vi "RunEntuse.vi"() -> ()   [LabVIEW 2012]
uses:
  <vilib>/addons/database/Connection.llb/DB Tools Open Connec (Path).vi
  <vilib>/addons/database/Connection.llb/Conn Execute.vi
  <vilib>/addons/database/Recordset.llb/Rec Fetch Recordset Data (R).vi
  <vilib>/addons/database/Recordset.llb/Rec Destroy - Connection.vi
  <vilib>/addons/database/Recordset.llb/Rec Fetch Integer Data (R).vi
  <vilib>/addons/database/_DB Variant To Data/Database Variant To Data.xnode
  <vilib>/addons/database/NI_Database_API.lvlib
panel:
  out "data 3":string
  out "data 2":string
  out "x > y?":bool
  out "concatenated string":string
  out "data":string
  out "error out":errorcluster
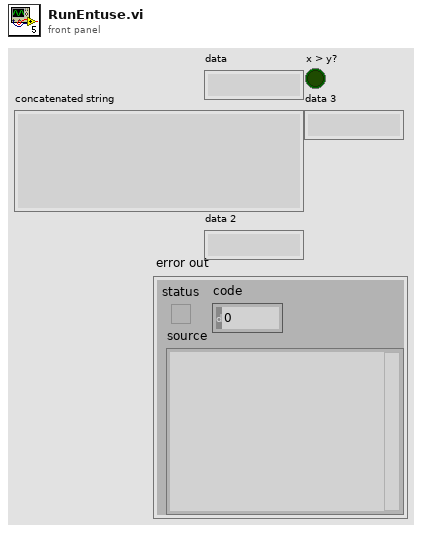
[diagram p1: front panel]
types:
  T1 = typedef "NI_Database_API.lvlib/Conn ObjectReference.ctl" = refnum<k1>
  T2 = typedef "NI_Database_API.lvlib/Rec ObjectReference.ctl" = refnum<k1>
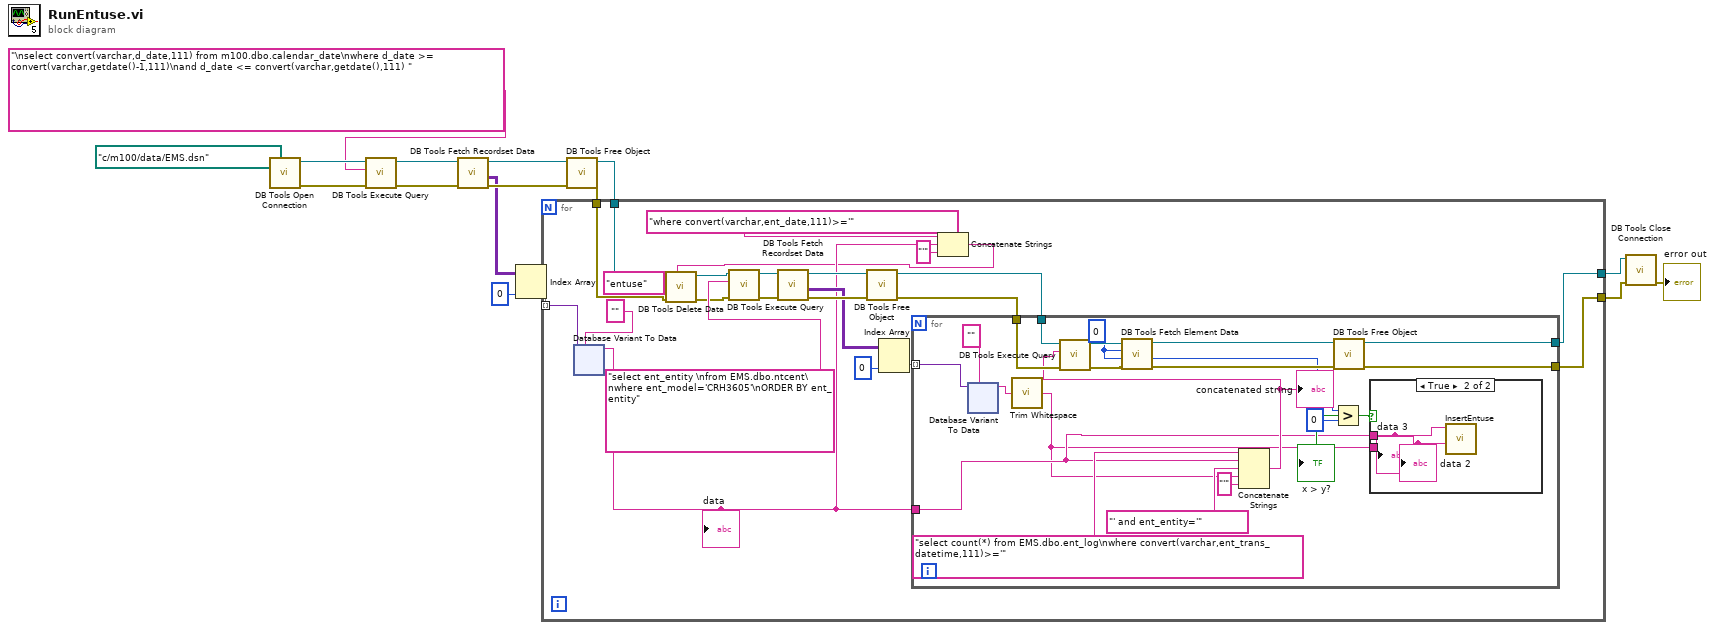
[diagram p0: block diagram]
diagram:
  n1 = call-poly <vilib>:"DB Tools Open Connection.vi"("connection information"=path "c:/m100/data/EMS.dsn") -> ("error out"=w12:errorcluster, "connection reference"=w15:T1)  [unwired: 7 in]
  n2 = call-poly <vilib>:"DB Tools Execute Query.vi"("error in (no error)"=w12, "SQL query"="\nselect convert(varchar,d_date,111) from m100.dbo.calendar_date\nwhere d_date >= convert(varchar,getdate()-1,111)\nand d_date <= convert(varchar,getdate(),111) " ("string"), "connection reference"=w15) -> ("error out"=w11:errorcluster, "recordset reference"=w14:T2)  [unwired: 5 in]
  n3 = call-poly <vilib>:"DB Tools Fetch Recordset Data.vi"("error in (no error)"=w11, "recordset reference"=w14) -> ("error out"=w10:errorcluster, "recordset data"=w7:variant[][], "recordset reference out"=w13:T2)  [unwired: 3 in]
  n4 = Index Array(array=w7, index (col)=0 ("disabled index (col)")) -> (element=w5:variant[])  [unwired: 1 in]
  n5 = call-poly <vilib>:"DB Tools Free Object.vi"("error in (no error)"=w10, "recordset reference"=w13) -> ("error out"=w3:errorcluster, "connection reference"=w4:T1)  [unwired: 8 in]
  n6 = for {
    tunnel: w5 -> [w39] mode=indexing
    tunnel: w4 -> [w23]
    tunnel: w3 -> [w22]
    tunnel: [w30] -> w2
    tunnel: [w29] -> w1
    n7 = xnode "Database Variant To Data"("database variant"=w39, "type"="") -> ("data"=w19:string)  [unwired: 1 in, 1 out]
    "data" <- w19
    n8 = Concatenate Strings("where convert(varchar,ent_date,111)>='" ("string"), w19, "'" ("string")) -> (w17:string)
    n9 = call <vilib>:"DB Tools Delete Data.vi"("condition"=w17, "error in (no error)"=w22, "table"="entuse", "connection reference"=w23) -> ("error out"=w24:errorcluster, "connection reference out"=w25:T1)  [unwired: 6 in]
    n10 = call-poly <vilib>:"DB Tools Execute Query.vi"("error in (no error)"=w24, "SQL query"="select ent_entity \nfrom EMS.dbo.ntcent\nwhere ent_model='CRH3605'\nORDER BY ent_entity" ("string"), "connection reference"=w25) -> ("error out"=w36:errorcluster, "recordset reference"=w38:T2)  [unwired: 5 in]
    n11 = call-poly <vilib>:"DB Tools Fetch Recordset Data.vi"("error in (no error)"=w36, "recordset reference"=w38) -> ("error out"=w35:errorcluster, "recordset data"=w33:variant[][], "recordset reference out"=w37:T2)  [unwired: 3 in]
    n12 = call-poly <vilib>:"DB Tools Free Object.vi"("error in (no error)"=w35, "recordset reference"=w37) -> ("error out"=w27:errorcluster, "connection reference"=w28:T1)  [unwired: 8 in]
    n13 = Index Array(array=w33, index (col)=0 ("disabled index (col)")) -> (element=w31:variant[])  [unwired: 1 in]
    n14 = for {
      tunnel: w31 -> [w60] mode=indexing
      tunnel: w19 -> [w42]
      tunnel: [w58] -> w30
      tunnel: [w57] -> w29
      tunnel: w28 -> [w52]
      tunnel: w27 -> [w51]
      w46 = 0
      n15 = xnode "Database Variant To Data"("database variant"=w60, "type"="") -> ("data"=w41:string)  [unwired: 1 in, 1 out]
      n16 = call <vilib>:"Trim Whitespace.vi"("string"=w41) -> ("trimmed string"=w40:string)  [unwired: 1 in]
      n17 = Concatenate Strings("select count(*) from EMS.dbo.ent_log\nwhere convert(varchar,ent_trans_datetime,111)>='" ("string"), w42, "' and ent_entity='" ("string"), w40, "'" ("string")) -> (w47:string)
      "concatenated string" <- w47
      n18 = call-poly <vilib>:"DB Tools Execute Query.vi"("error in (no error)"=w51, "SQL query"=w47, "connection reference"=w52) -> ("error out"=w53:errorcluster, "recordset reference"=w54:T2)  [unwired: 5 in]
      n19 = call-poly <vilib>:"DB Tools Fetch Element Data.vi"("error in (no error)"=w53, "type"=w46, "column index"=w46, "recordset reference"=w54) -> ("error out"=w55:errorcluster, "data"=w45:i32, "recordset reference out"=w56:T2)  [unwired: 3 in]
      n20 = Greater?(x=w45, y=0) -> (0:w43:bool)
      "x > y?" <- w43
      n21 = call-poly <vilib>:"DB Tools Free Object.vi"("error in (no error)"=w55, "recordset reference"=w56) -> ("error out"=w57:errorcluster, "connection reference"=w58:T1)  [unwired: 8 in]
      n22 = case shown="True" w43 {
        tunnel: w42 -> [_ w62]
        tunnel: w40 -> [_ w61]
        frame False {
        }
        frame True {
          n23 = call "InsertEntuse.vi"("Entity"=w61, "Date"=w62) -> ()  [unwired: 10 in]
          "data 2" <- w61
          "data 3" <- w62
        }
      }
    }
  }
  n24 = call <vilib>:"DB Tools Close Connection.vi"("error in (no error)"=w1, "connection reference"=w2) -> ("error out"=→"error out":errorcluster)  [unwired: 5 in]
